vi "LVPortMakeObjectMapNamepthData.vi"(8 "Labview Contriner type":T1, 9 "value":variant, 10 "name":string, 11 "MatlabType":T3) -> (3 "MatlabDataBundle":T2)   [LabVIEW 2017]
uses:
  LVPortObjectMapDataTypeEnum.ctl
  LVPortObjectMapNamepathData.ctl
  LVPortObjectMapContainerTypeEnum.ctl
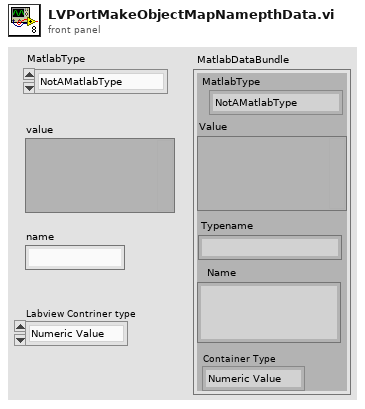
[diagram p1: front panel]
types:
  T1 = typedef "LVPortObjectMapContainerTypeEnum.ctl" = enum16{"Numeric Value", "Numeric Array", "Waveform"}
  T2 = typedef "LVPortObjectMapNamepathData.ctl" = cluster{"MatlabType":T3, "Value":variant, "Name":string, "Typename":string, "Container Type":T1}
  T3 = typedef "LVPortObjectMapDataTypeEnum.ctl" = enum16{"NotAMatlabType", "Real", "Complex", "String", "Boolean"}
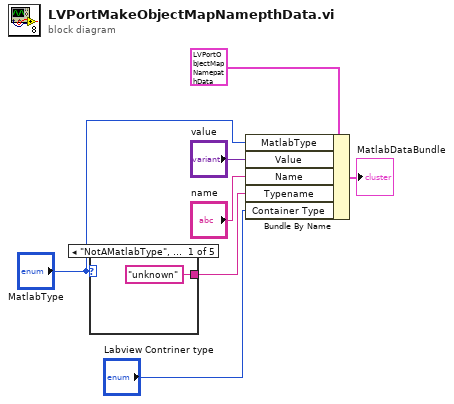
[diagram p0: block diagram]
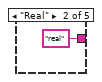
[diagram p2: hidden frame]
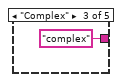
[diagram p3: hidden frame]
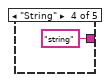
[diagram p4: hidden frame]
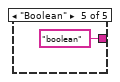
[diagram p5: hidden frame]
diagram:
  n1 = case shown="\"NotAMatlabType\", Default" "MatlabType" {
    tunnel: ["unknown" ("Typename") "real" ("Typename") "complex" ("Typename") "string" ("Typename") "boolean" ("Typename")] -> w2
    frame "NotAMatlabType", Default {
    }
    frame "Real" {
    }
    frame "Complex" {
    }
    frame "String" {
    }
    frame "Boolean" {
    }
  }
  n2 = Bundle By Name(cluster=T2 {"MatlabType"=enum."NotAMatlabType", "Value"=variant, "Name"="", "Typename"="", "Container Type"=enum."Numeric Value"} ("input cluster"), "MatlabType"="MatlabType", "Value"="value", "Name"="name", "Typename"=w2, "Container Type"="Labview Contriner type") -> (→"MatlabDataBundle":T2)
